vi "Demo.vi"() -> ()   [LabVIEW 2018]
panel:
  out "Boolean 2":bool
  out "Boolean":bool
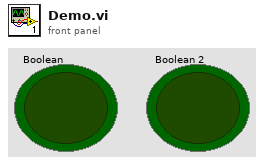
[diagram p1: front panel]
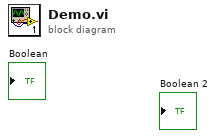
[diagram p0: block diagram]
diagram:
